vi "AWS-S3-ProcessDownload.vi"(0 "Get Object Response":refnum<k24>, 5 "Download Complete Event":refnum<user-event>, 7 "Destination Path (Local)":path, 11 "error in":errorcluster) -> ()   [LabVIEW 2012, in "AWS-S3-API.lvclass"]
uses:
  AWS-S3-API.lvclass
  C:/Users/Jack/repo/aws/AWS-SDK/AWSSDK.dll
  repo/aws/AWS-SDK/AWSSDK.dll
  AWS-S3-Transfer-Header.ctl
  AWS-S3-Transfer-Completed.ctl
panel:
  # "Inputs"
  # "Outputs"
  # "No Outputs - this VI\nis fire and forget"
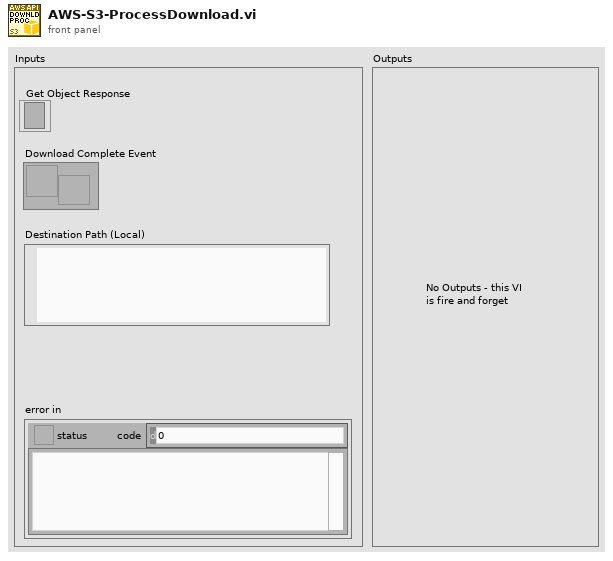
[diagram p1: front panel]
types:
  T1 = typedef "AWS-S3-API.lvclass/AWS-S3-Transfer-Completed.ctl" = cluster{"Transfer Header":T2, "Error?":bool, "Error Message":string}
  T2 = typedef "AWS-S3-API.lvclass/AWS-S3-Transfer-Header.ctl" = cluster{"Bucket Name":string, "Object Name":string, "Local Filepath":path}
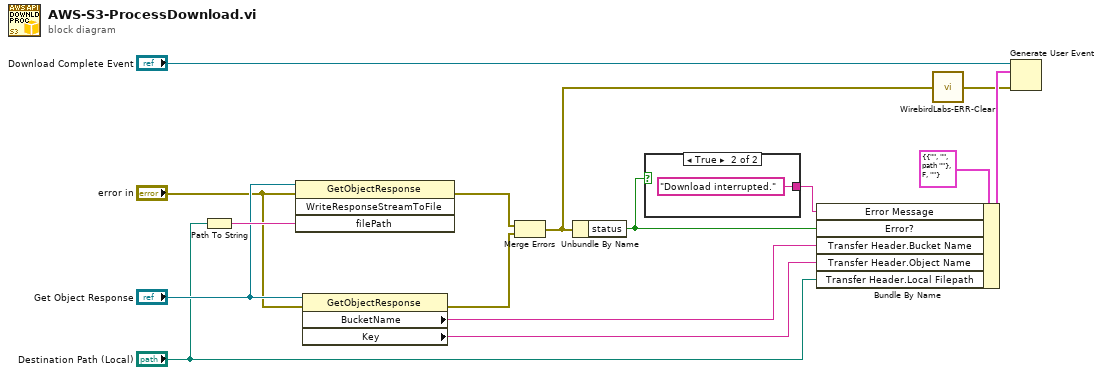
[diagram p0: block diagram]
diagram:
  n1 = Path To String(path="Destination Path (Local)") -> (string=w15:string)
  n2 = invoke class="GetObjectResponse" method="WriteResponseStreamToFile"(reference="Get Object Response", error in="error in", "filePath"=w15) -> (error out=w5:errorcluster)  [unwired: 1 in, 3 out]
  n3 = property class="GetObjectResponse"(reference="Get Object Response", error in="error in") -> (error out=w6:errorcluster, "BucketName"=w9:string, "Key"=w8:string)  [unwired: 1 out]
  n4 = Merge Errors(w5, w6) -> (w4:errorcluster)
  n5 = Unbundle By Name(w4) -> ("status"=w2:bool)
  n6 = case shown="True" w2 {
    tunnel: [_ "Download interrupted." ("source")] -> w1
    frame False {
    }
    frame True {
    }
  }
  n7 = Bundle By Name(cluster=T1 {"Transfer Header"={"Bucket Name"="", "Object Name"="", "Local Filepath"=path ""}, "Error?"=FALSE, "Error Message"=""}, "Error Message"=w1, "Error?"=w2, "Transfer Header.Bucket Name"=w9, "Transfer Header.Object Name"=w8, "Transfer Header.Local Filepath"="Destination Path (Local)") -> (w12:T1)
  n8 = call "WirebirdLabs-ERR-Clear.vi"("error to snuff"=w4) -> ("no error"=w3:errorcluster)
  n9 = Generate User Event(user event="Download Complete Event", event data cluster=w12, error in=w3) -> ()  [unwired: 2 out]
